vi "Clear Map.vi"(0 "DBMap in":refnum<class "DBMap.lvclass">, 11 "error in (no error)":errorcluster {"code" format="Error %.0f"}) -> (4 "DBMap out":refnum<class "DBMap.lvclass">, 15 "error out":errorcluster {"code" format="Error %.0f"})   [LabVIEW 2020, in "DBMap.lvclass"]
uses:
  DBMap.lvclass
  DBMap.lvclass/DBMap.ctl
  <vilib>/drjdpowell/SQLite Library/SQLite.lvlib
  <vilib>/drjdpowell/SQLite Library/SQL Connection/Execute SQL (No results).vi
  <vilib>/drjdpowell/SQLite Library/SQL Connection/Connection.lvclass
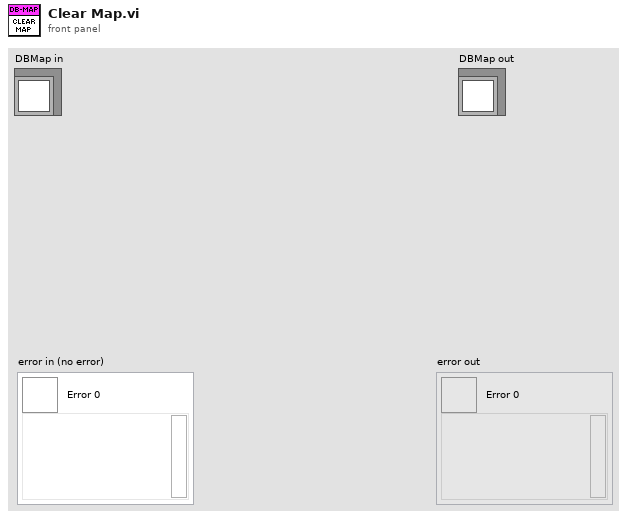
[diagram p1: front panel]
types:
  T1 = typedef "Semaphore RefNum" = refnum<k1>
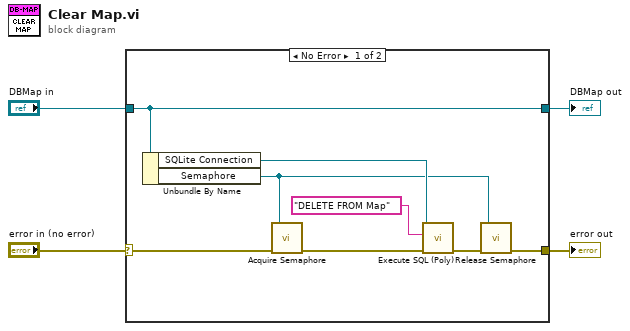
[diagram p0: block diagram]
diagram:
  n1 = case shown="No Error" "error in (no error)" {
    selector: "error in (no error)" -> [w11 w14]
    tunnel: [w6 w14] -> w3
    tunnel: [w12 w13] -> w1
    tunnel: "DBMap in" -> [w12 w13]
    frame No Error {
      n2 = Unbundle By Name(w12) -> ("SQLite Connection"=w8:refnum<class "Connection.lvclass">, "Semaphore"=w5:T1)
      n3 = call <vilib>:"Acquire Semaphore.vi"("error in (no error)"=w11, "semaphore"=w5) -> ("error out"=w9:errorcluster)  [unwired: 3 in, 2 out]
      n4 = call-poly <vilib>:"Execute SQL (Poly).vi"("error in (no error)"=w9, "SQL"="DELETE FROM Map", "SQLite Connection in"=w8) -> ("error out"=w7:errorcluster)  [unwired: 7 in, 1 out]
      n5 = call <vilib>:"Release Semaphore.vi"("error in (no error)"=w7, "semaphore"=w5) -> ("error out"=w6:errorcluster)  [unwired: 4 in, 1 out]
    }
    frame Error {
    }
  }
  "error out" <- w3
  "DBMap out" <- w1
